vi "20154187-许立锐-车型识别.vi"() -> ()   [LabVIEW 2012]
uses:
  <vilib>/Utility/file.llb/Write To Spreadsheet File (string).vi
  <vilib>/vision/NI_Vision_Development_Module.lvlib
panel:
  out "结果值":i32
  out "货车":bool
  out "面包车":bool
  out "轿车":bool
  out "客车":bool
  out "Roof_Midpoint":dbl
  out "Rear_Botton":i32
  out "Front_Botton":i32
  out "Front_Roof":i32
  out "X_Right":i32
  out "Y_Bottom":i32
  out "Y_Roof":i32
  out "X_Left":i32
  in  "处理结果":enum32{"图像处理", "车型判断"}(tab)
  out "原图":T1(plugin-control)
  out "差分图":T1(plugin-control)
  out "二值图":T1(plugin-control)
  out "闭操作结果":T1(plugin-control)
  out "填充图":T1(plugin-control)
  out "图像裁剪":T1(plugin-control)
  in  "车辆图":path
  out "车型判断结果":string
  out "Height1":i32
  out "Front/Rear":dbl
  out "Roof/Botton":dbl
  out "Botton_Length":i32
  out "Roof_Length":i32
  out "Heighe2":i32
  out "Roof_Left":i32
  out "Roof_Right":i32
  out "Botton_Left":i32
  out "Botton_Right":i32
  out "车头列":u8[](array[numeric])
  out "车尾列":u8[](array[numeric])
  out "车顶行":u8[](array[numeric])
  out "车底行":u8[](array[numeric])
  out "Rear_Roof":i32
  out "Roof_Position":dbl
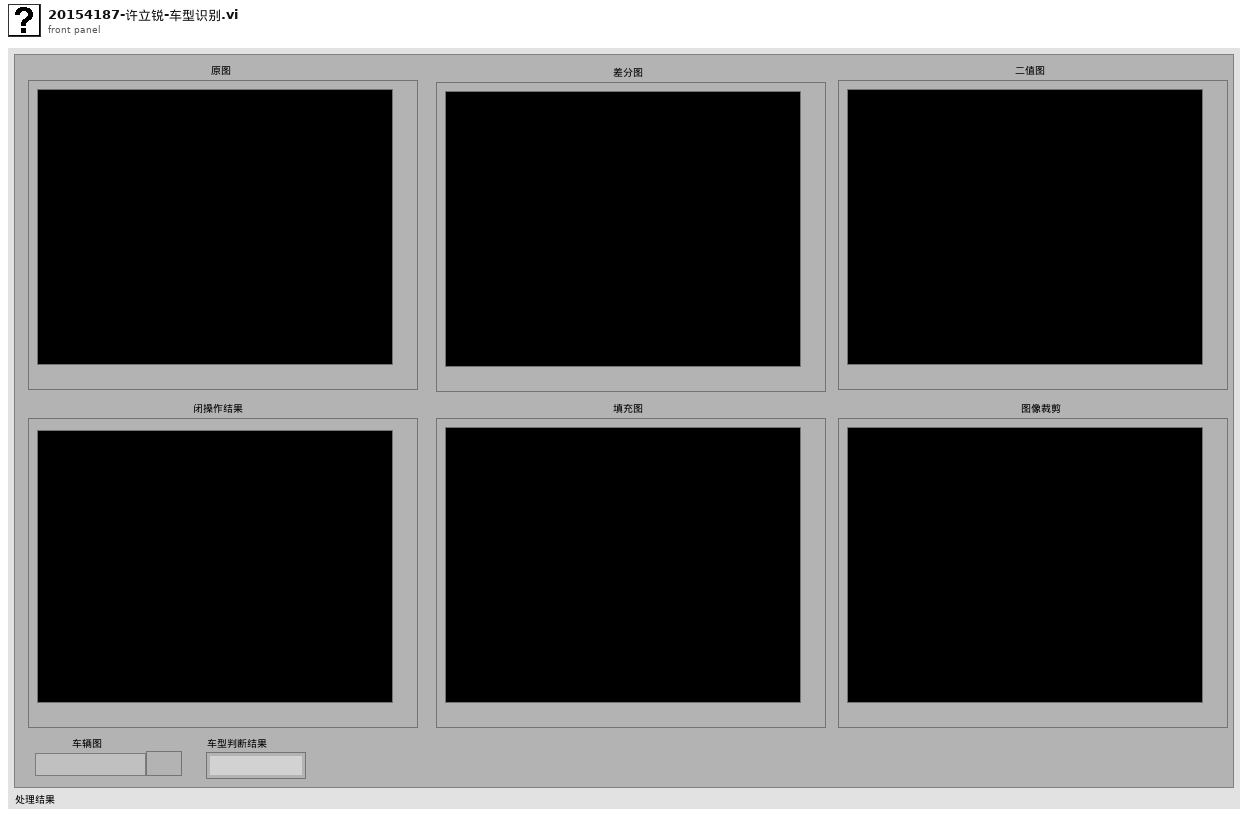
[diagram p1: front panel]
types:
  T1 = typedef "IMAQ Image.ctl" = refnum<image>
  T2 = typedef "Image Type" = u32
  T3 = typedef "imagedata.ctl" = cluster{"image type":i32, "image depth":i32, "image":u8[], "mask":u8[], "colors":u32[], "Rectangle":cluster{"left":i16, "top":i16, "right":i16, "bottom":i16}}
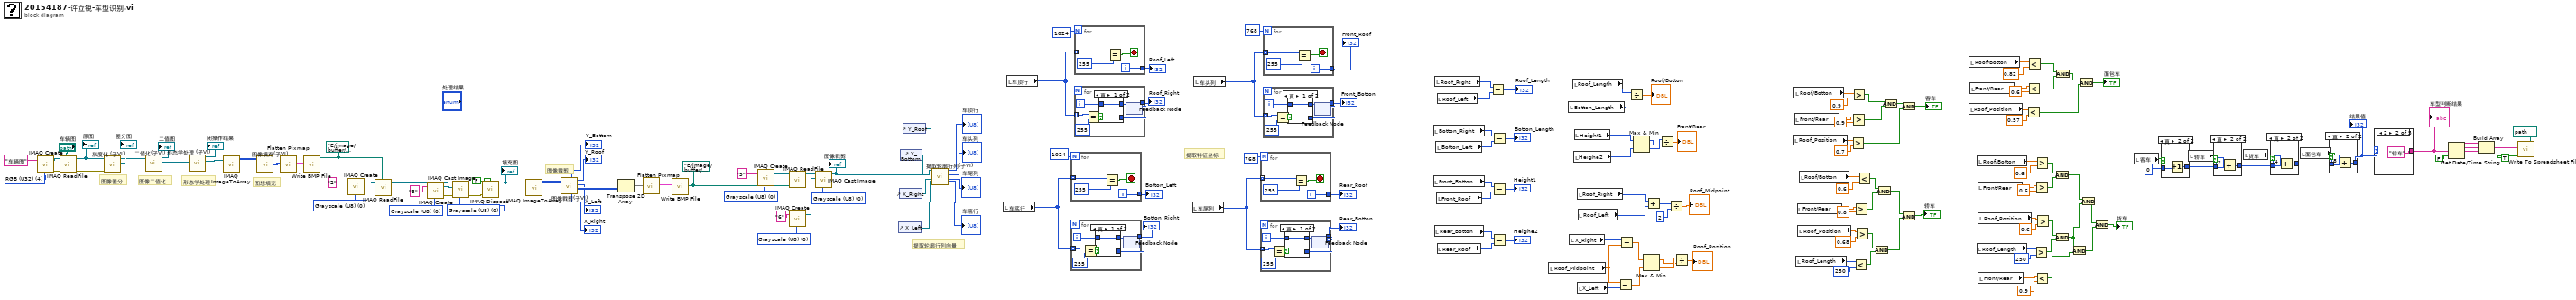
[diagram p0: block diagram]
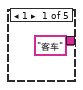
[diagram p6: hidden frame]
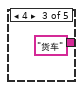
[diagram p7: hidden frame]
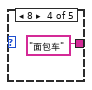
[diagram p8: hidden frame]
diagram:
  w1 = T2 4 items=["Grayscale (U8)", "Grayscale (I16)", "Grayscale (SGL)", "Complex (CSG)", "RGB (U32)", "HSL (U32)", "RGB (U64)", "Grayscale (U16)"] ("Image Type")
  w155 = T2 0 items=["Grayscale (U8)", "Grayscale (I16)", "Grayscale (SGL)", "Complex (CSG)", "RGB (U32)", "HSL (U32)", "RGB (U64)", "Grayscale (U16)"] ("Image Type")
  w157 = T2 0 items=["Grayscale (U8)", "Grayscale (I16)", "Grayscale (SGL)", "Complex (CSG)", "RGB (U32)", "HSL (U32)", "RGB (U64)", "Grayscale (U16)"] ("Image Type")
  w160 = T2 0 items=["Grayscale (U8)", "Grayscale (I16)", "Grayscale (SGL)", "Complex (CSG)", "RGB (U32)", "HSL (U32)", "RGB (U64)", "Grayscale (U16)"] ("Image Type")
  w177 = path "E:/image/buffer/afterClipping.bmp" ("path to BMP file")
  w167 = T2 0 items=["Grayscale (U8)", "Grayscale (I16)", "Grayscale (SGL)", "Complex (CSG)", "RGB (U32)", "HSL (U32)", "RGB (U64)", "Grayscale (U16)"] ("Image Type")
  w169 = T2 0 items=["Grayscale (U8)", "Grayscale (I16)", "Grayscale (SGL)", "Complex (CSG)", "RGB (U32)", "HSL (U32)", "RGB (U64)", "Grayscale (U16)"] ("Image Type")
  w172 = T2 0 items=["Grayscale (U8)", "Grayscale (I16)", "Grayscale (SGL)", "Complex (CSG)", "RGB (U32)", "HSL (U32)", "RGB (U64)", "Grayscale (U16)"] ("Image Type")
  w39 = path "E:/image/buffer/afterfilling.bmp" ("path to JPEG file")
  # "提取轮廓行列向量"
  # "图像裁剪"
  # "图想填充"
  # "形态学处理"
  # "图像二值化"
  # "图像差分"
  # "提取特征坐标"
  n1 = call "IMAQ Create"("Image Name"="车辆图", "Image Type"=w1) -> ("New Image"=w37:T1, "error out"=w35:errorcluster)  [unwired: 3 in]
  n2 = call "IMAQ ReadFile"("File Path"="车辆图", "error in (no error)"=w35, "Image"=w37) -> ("error out"=w25:errorcluster, "Image Out"=w26:T1)  [unwired: 4 in, 3 out]
  "原图" <- w26
  n3 = call "灰度化 (子VI).vi"("错误输入（无错误）"=w25, "引用句柄输入"=w26) -> ("图像差分"=→"差分图":T1, "引用句柄输出"=w19:T1)  [unwired: 7 in, 1 out]
  n4 = call "二值化(子VI).vi"("引用句柄输入"=w19) -> ("Image Dst Out"=w23:T1, "引用句柄输出"=→"二值图":T1)  [unwired: 9 in]
  n5 = call "形态学处理 (子VI).vi"("引用句柄输入"=w23) -> ("Image Dst Out"=w22:T1, "引用句柄输出"=→"闭操作结果":T1)  [unwired: 9 in]
  n6 = call "IMAQ ImageToArray"("Image"=w22) -> ("Image Pixels (U8)"=w20:u8[][])  [unwired: 3 in, 4 out]
  n7 = call "图像填充(子VI).vi"("Image Pixels (U8)"=w20) -> ("数组"=w174:u8[][])  [unwired: 10 in]
  n8 = call <vilib>:"Flatten Pixmap.vi"("8-bit pixmap"=w174) -> ("image data"=w175:T3)  [unwired: 10 in]
  n9 = call <vilib>:"Write BMP File.vi"("image data"=w175, "path to BMP file"=w39) -> ()  [unwired: 8 in, 2 out]
  n10 = call "IMAQ Create"("Image Name"="2", "Image Type"=w172) -> ("New Image"=w173:T1)  [unwired: 3 in, 1 out]
  n11 = call "IMAQ ReadFile"("File Path"=w39, "Image"=w173) -> ("Image Out"=w166:T1)  [unwired: 5 in, 4 out]
  n12 = call "IMAQ Create"("Image Name"="3", "Image Type"=w169) -> ("New Image"=w168:T1, "error out"=w34:errorcluster)  [unwired: 3 in]
  n13 = call "IMAQ Cast Image"("Image Type"=w167, "error in (no error)"=w34, "Image Dst"=w168, "Image Src"=w166) -> ("error out"=w33:errorcluster, "Image Dst Out"=w2:T1)  [unwired: 6 in]
  "填充图" <- w2
  n14 = call "IMAQ Dispose"("All Images? (No)"=FALSE, "error in (no error)"=w33) -> ()  [unwired: 4 in, 1 out]
  n15 = call "IMAQ ImageToArray"("Image"=w2) -> ("Image Pixels (U8)"=w165:u8[][])  [unwired: 3 in, 4 out]
  n16 = call "图像裁剪(子VI).vi"("Image Pixels (U8)"=w165) -> ("数组"=w164:u8[][], "X_Left"=→"X_Left":i32, "Y_Roof"=→"Y_Roof":i32, "X_Right"=→"X_Right":i32, "Y_Bottom"=→"Y_Bottom":i32)  [unwired: 6 in]
  n17 = Transpose 2D Array(2D array=w164) -> (transposed array=w163:u8[][])
  n18 = call <vilib>:"Flatten Pixmap.vi"("8-bit pixmap"=w163) -> ("image data"=w162:T3)  [unwired: 10 in]
  n19 = call <vilib>:"Write BMP File.vi"("image data"=w162, "path to BMP file"=w177) -> ()  [unwired: 8 in, 2 out]
  n20 = call "IMAQ Create"("Image Name"="5", "Image Type"=w160) -> ("New Image"=w161:T1)  [unwired: 3 in, 1 out]
  n21 = call "IMAQ ReadFile"("File Path"=w177, "Image"=w161) -> ("Image Out"=w154:T1)  [unwired: 5 in, 4 out]
  n22 = call "IMAQ Create"("Image Name"="6", "Image Type"=w157) -> ("New Image"=w156:T1)  [unwired: 3 in, 1 out]
  n23 = call "IMAQ Cast Image"("Image Type"=w155, "Image Dst"=w156, "Image Src"=w154) -> ("Image Dst Out"=w176:T1)  [unwired: 7 in, 1 out]
  "图像裁剪" <- w176
  n24 = control-ref of="X_Left"() -> (w15:refnum<vi>)
  n25 = control-ref of="X_Right"() -> (w16:refnum<vi>)
  n26 = control-ref of="Y_Bottom"() -> (w17:refnum<vi>)
  n27 = control-ref of="Y_Roof"() -> (w18:refnum<vi>)
  n28 = call "提取轮廓行列(子VI).vi"("reference 3"=w15, "reference"=w18, "reference 4"=w16, "reference 2"=w17, "引用句柄输入"=w176) -> ("车尾列"=→"车尾列":u8[], "车头列"=→"车头列":u8[], "车顶行"=→"车顶行":u8[], "车底行"=→"车底行":u8[])  [unwired: 3 in]
  n29 = local read "车底行"() -> (w150:u8[])
  n30 = local read "车顶行"() -> (w152:u8[])
  n31 = for {
    N: 1024 -> [_]
    tunnel: w150 -> [w179] mode=indexing
    tunnel: [w178] -> w144
    i -> [w178]
    stop <- w180 stop-if-true
    n32 = Equal?(x=w179, y=u8 255) -> (x = y?=w180:bool)
  }
  "Botton_Left" <- w144
  n33 = for {
    tunnel: w150 -> [w183] mode=indexing
    tunnel: [w185] -> w141
    i -> [w187]
    n34 = Equal?(x=w183, y=u8 255) -> (x = y?=w184:bool)
    n35 = feedback #1() -> (w185:i32)  [unwired: 1 in]
    n36 = case shown="真" w184 {
      tunnel: w187 -> [w188 _]
      tunnel: [w188 w189] -> w186
      tunnel: w185 -> [_ w189]
      frame True {
      }
      frame False {
      }
    }
    n37 = feedback-in #1(w186) -> ()
  }
  "Botton_Right" <- w141
  n38 = for {
    N: 1024 -> [_]
    tunnel: w152 -> [w191] mode=indexing
    tunnel: [w190] -> w145
    i -> [w190]
    stop <- w192 stop-if-true
    n39 = Equal?(x=w191, y=u8 255) -> (x = y?=w192:bool)
  }
  "Roof_Left" <- w145
  n40 = for {
    tunnel: w152 -> [w195] mode=indexing
    tunnel: [w197] -> w142
    i -> [w199]
    n41 = Equal?(x=w195, y=u8 255) -> (x = y?=w196:bool)
    n42 = feedback #2() -> (w197:i32)  [unwired: 1 in]
    n43 = case shown="真" w196 {
      tunnel: w199 -> [w200 _]
      tunnel: [w200 w201] -> w198
      tunnel: w197 -> [_ w201]
      frame True {
      }
      frame False {
      }
    }
    n44 = feedback-in #2(w198) -> ()
  }
  "Roof_Right" <- w142
  n45 = local read "车尾列"() -> (w149:u8[])
  n46 = local read "车头列"() -> (w147:u8[])
  n47 = for {
    N: 768 -> [_]
    tunnel: w149 -> [w203] mode=indexing
    tunnel: [w202] -> w139
    i -> [w202]
    stop <- w204 stop-if-true
    n48 = Equal?(x=w203, y=u8 255) -> (x = y?=w204:bool)
  }
  "Rear_Roof" <- w139
  n49 = for {
    tunnel: w149 -> [w208] mode=indexing
    tunnel: [w206] -> w138
    tunnel: [w206] -> _ mode=indexing
    i -> [w211]
    n50 = Equal?(x=w208, y=u8 255) -> (x = y?=w209:bool)
    n51 = feedback #3() -> (w206:i32)  [unwired: 1 in]
    n52 = case shown="真" w209 {
      tunnel: w211 -> [w212 _]
      tunnel: [w212 w213] -> w210
      tunnel: w206 -> [_ w213]
      frame True {
      }
      frame False {
      }
    }
    n53 = feedback-in #3(w210) -> ()
  }
  "Rear_Botton" <- w138
  n54 = for {
    N: 768 -> [_]
    tunnel: w147 -> [w215] mode=indexing
    tunnel: [w214] -> w140
    i -> [w214]
    stop <- w216 stop-if-true
    n55 = Equal?(x=w215, y=u8 255) -> (x = y?=w216:bool)
  }
  "Front_Roof" <- w140
  n56 = for {
    tunnel: w147 -> [w219] mode=indexing
    tunnel: [w221] -> w143
    i -> [w223]
    n57 = Equal?(x=w219, y=u8 255) -> (x = y?=w220:bool)
    n58 = feedback #4() -> (w221:i32)  [unwired: 1 in]
    n59 = case shown="真" w220 {
      tunnel: w223 -> [w224 _]
      tunnel: [w224 w225] -> w222
      tunnel: w221 -> [_ w225]
      frame True {
      }
      frame False {
      }
    }
    n60 = feedback-in #4(w222) -> ()
  }
  "Front_Botton" <- w143
  n61 = local read "Botton_Right"() -> (w135:i32)
  n62 = local read "Front_Botton"() -> (w133:i32)
  n63 = local read "Rear_Botton"() -> (w132:i32)
  n64 = local read "Roof_Right"() -> (w137:i32)
  n65 = local read "Botton_Left"() -> (w134:i32)
  n66 = local read "Front_Roof"() -> (w130:i32)
  n67 = local read "Roof_Left"() -> (w136:i32)
  n68 = local read "Rear_Roof"() -> (w131:i32)
  n69 = Subtract(x=w137, y=w136) -> (x-y=→"Roof_Length":i32)
  n70 = Subtract(x=w135, y=w134) -> (x-y=→"Botton_Length":i32)
  n71 = Subtract(x=w133, y=w130) -> (x-y=→"Height1":i32)
  n72 = Subtract(x=w132, y=w131) -> (x-y=→"Heighe2":i32)
  n73 = local read "Roof_Midpoint"() -> (w111:dbl)
  n74 = local read "Botton_Length"() -> (w124:i32)
  n75 = local read "X_Right"() -> (w112:i32)
  n76 = local read "Roof_Length"() -> (w125:i32)
  n77 = local read "Heighe2"() -> (w121:i32)
  n78 = local read "Height1"() -> (w122:i32)
  n79 = local read "Roof_Right"() -> (w117:i32)
  n80 = local read "X_Left"() -> (w110:i32)
  n81 = local read "Roof_Left"() -> (w116:i32)
  n82 = Subtract(x=w111, y=w110) -> (x-y=w108:dbl)
  n83 = Subtract(x=w112, y=w111) -> (x-y=w109:dbl)
  n84 = Divide(x=w125, y=w124) -> (x/y=→"Roof/Botton":dbl)
  n85 = Max & Min(x=w122, y=w121) -> (max(x,y)=w119:i32, min(x,y)=w120:i32)
  n86 = Max & Min(x=w109, y=w108) -> (max(x,y)=w99:dbl, min(x,y)=w100:dbl)
  n87 = Add(x=w117, y=w116) -> (x+y=w115:i32)
  n88 = Divide(x=w120, y=w119) -> (x/y=→"Front/Rear":dbl)
  n89 = Divide(x=w115, y=2) -> (x/y=→"Roof_Midpoint":dbl)
  n90 = Divide(x=w100, y=w99) -> (x/y=→"Roof_Position":dbl)
  n91 = local read "Roof_Position"() -> (w102:dbl)
  n92 = local read "Roof/Botton"() -> (w106:dbl)
  n93 = local read "Front/Rear"() -> (w104:dbl)
  n94 = local read "Roof_Length"() -> (w87:i32)
  n95 = local read "Front/Rear"() -> (w90:dbl)
  n96 = local read "Roof_Position"() -> (w92:dbl)
  n97 = local read "Roof/Botton"() -> (w88:dbl)
  n98 = Greater?(x=w102, y=0.7) -> (0:w96:bool)
  n99 = Greater?(x=w104, y=0.9) -> (0:w97:bool)
  n100 = Greater?(x=w106, y=0.9) -> (0:w98:bool)
  n101 = Less?(x=w87, y=250) -> (x < y?=w82:bool)
  n102 = Greater?(x=w90, y=0.8) -> (0:w84:bool)
  n103 = Greater?(x=w92, y=0.68) -> (0:w83:bool)
  n104 = Less?(x=w88, y=0.6) -> (x < y?=w85:bool)
  n105 = And(x=w83, y=w82) -> (x .and. y?=w81:bool)
  n106 = And(x=w85, y=w84) -> (x .and. y?=w80:bool)
  n107 = And(x=w98, y=w97) -> (x .and. y?=w95:bool)
  n108 = And(x=w95, y=w96) -> (x .and. y?=→"客车":bool)
  n109 = And(x=w80, y=w81) -> (x .and. y?=→"轿车":bool)
  n110 = local read "Roof_Position"() -> (w77:dbl)
  n111 = local read "Roof/Botton"() -> (w73:dbl)
  n112 = local read "Front/Rear"() -> (w75:dbl)
  n113 = local read "Roof_Length"() -> (w61:i32)
  n114 = local read "Roof/Botton"() -> (w60:dbl)
  n115 = local read "Front/Rear"() -> (w58:dbl)
  n116 = local read "Roof_Position"() -> (w56:dbl)
  n117 = local read "Front/Rear"() -> (w44:dbl)
  n118 = Less?(x=w77, y=0.57) -> (x < y?=w69:bool)
  n119 = Less?(x=w75, y=0.6) -> (x < y?=w70:bool)
  n120 = Less?(x=w73, y=0.82) -> (x < y?=w71:bool)
  n121 = Greater?(x=w61, y=250) -> (0:w66:bool)
  n122 = Greater?(x=w58, y=0.6) -> (0:w64:bool)
  n123 = Greater?(x=w60, y=0.6) -> (0:w63:bool)
  n124 = Less?(x=w44, y=0.9) -> (x < y?=w42:bool)
  n125 = Greater?(x=w56, y=0.6) -> (0:w65:bool)
  n126 = And(x=w63, y=w64) -> (x .and. y?=w67:bool)
  n127 = And(x=w65, y=w66) -> (x .and. y?=w43:bool)
  n128 = And(x=w71, y=w70) -> (x .and. y?=w72:bool)
  n129 = And(x=w43, y=w42) -> (x .and. y?=w10:bool)
  n130 = And(x=w72, y=w69) -> (x .and. y?=→"面包车":bool)
  n131 = And(x=w67, y=w43) -> (x .and. y?=w41:bool)
  n132 = And(x=w41, y=w10) -> (x .and. y?=→"货车":bool)
  n133 = local read "客车"() -> (w54:bool)
  n134 = case shown="真" w54 {
    tunnel: 0 -> [w226 w228]
    tunnel: [w226 w227] -> w51
    frame False {
    }
    frame True {
      n135 = Increment(x=w228) -> (x+1=w227:i32)
    }
  }
  n136 = local read "轿车"() -> (w52:bool)
  n137 = case shown="真" w52 {
    tunnel: w51 -> [w229 w232]
    tunnel: [w229 w231] -> w49
    frame False {
    }
    frame True {
      n138 = Add(x=2, y=w232) -> (x+y=w231:i32)
    }
  }
  n139 = local read "货车"() -> (w50:bool)
  n140 = case shown="真" w50 {
    tunnel: w49 -> [w233 w236]
    tunnel: [w233 w235] -> w47
    frame False {
    }
    frame True {
      n141 = Add(x=4, y=w236) -> (x+y=w235:i32)
    }
  }
  n142 = local read "面包车"() -> (w48:bool)
  n143 = case shown="真" w48 {
    tunnel: w47 -> [w237 w240]
    tunnel: [w237 w239] -> w46
    frame False {
    }
    frame True {
      n144 = Add(x=8, y=w240) -> (x+y=w239:i32)
    }
  }
  "结果值" <- w46
  n145 = case shown="2" w46 {
    tunnel: ["客车" "轿车" "货车" "面包车" _] -> w3
    frame 1 {
    }
    frame 2 {
    }
    frame 4 {
    }
    frame 8 {
    }
    frame Default {
    }
  }
  "车型判断结果" <- w3
  n146 = Get Date/Time String(want seconds? (F)=FALSE ("需要秒？(F)")) -> (date string=w9:string, time string=w8:string)  [unwired: 2 in]
  n147 = Build Array(w9, w8, w3) -> (w6:string[])
  n148 = call-poly <vilib>:"Write To Spreadsheet File.vi"("append to file? (new file:F)"=TRUE, "1D data"=w6, "file path (dialog if empty)"=path "E:/image/buffer/历史数据.txt") -> ()  [unwired: 5 in, 1 out]
